vi "Hex to Decimal(SubVI).vi"(11 "String in":string) -> (3 "Array":u32[][](array[numeric]))   [LabVIEW 2017]
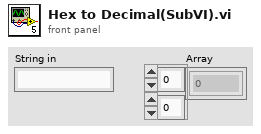
[diagram p1: front panel]
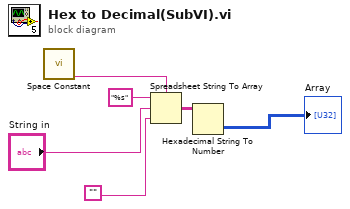
[diagram p0: block diagram]
diagram:
  n1 = call <vilib>:"Space Constant.vi"() -> ("String"=w2:string)
  n2 = Spreadsheet String To Array(delimiter (Tab)=w2, format string="%s" ("spreadsheet string"), spreadsheet string="String in", array type (2D Dbl)="") -> (array=w5:string[][])
  n3 = Hexadecimal String To Number(string=w5) -> (number=→"Array":u32[][])  [unwired: 2 in, 1 out]
